vi "enable motors.vi"(8 "error in (no error)":errorcluster) -> (0 "error out":errorcluster, 3 "function return":i32)   [LabVIEW 2014, in "libroboticscape.lvlib"]
doc: "int enable_motors();"
uses:
  libroboticscape.lvlib
  <vilib>/wsapi/NI_WebServices.lvlib
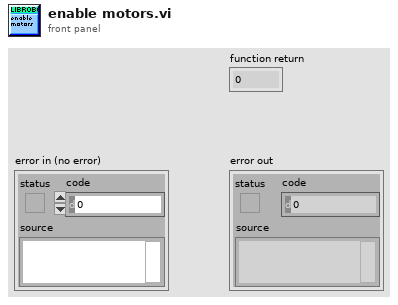
[diagram p1: front panel]
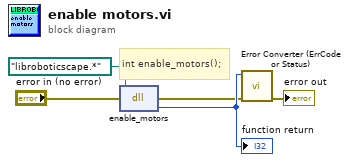
[diagram p0: block diagram]
diagram:
  # "int enable_motors();"
  n1 = dll-call lib="C:/Users/ktalke/Documents/Jessie Build/Libroboticscape/libroboticscape.so" fn="enable_motors"(path in=path "libroboticscape.*", error in="error in (no error)") -> (error out=w3:errorcluster, "return type"=w5:i32)  [unwired: 1 in, 1 out]
  "function return" <- w5
  n2 = call <vilib>:"Error Converter (ErrCode or Status).vi"("error in (no error)"=w3, "error code"=w5) -> ("error out"=→"error out":errorcluster)  [unwired: 9 in]
